vi "Obtain Doc Win ID.vi"(8 "error in (no error)":errorcluster, 11 "Document in":refnum<class "Document.lvclass">) -> (0 "error out":errorcluster, 3 "Document out":refnum<class "Document.lvclass">)   [LabVIEW 2016, in "Document.lvclass"]
uses:
  Document.lvclass
  Document.lvclass/Document.ctl
  user32.dll
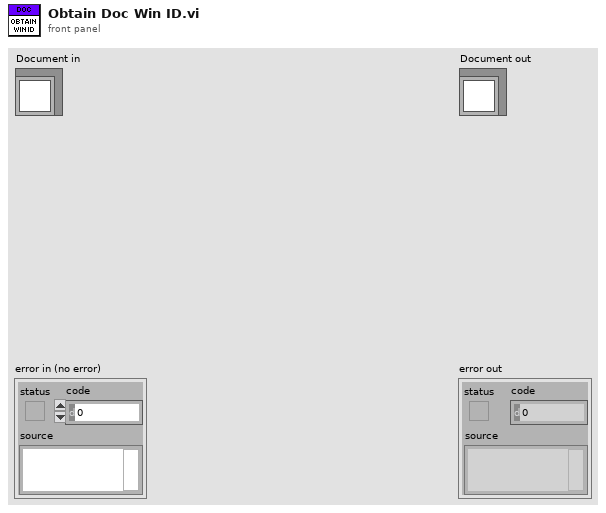
[diagram p1: front panel]
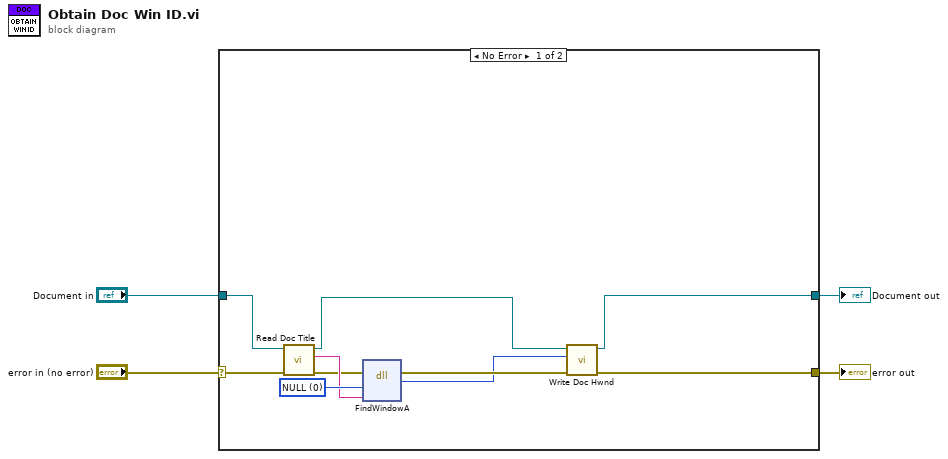
[diagram p0: block diagram]
diagram:
  n1 = case shown="No Error" "error in (no error)" {
    selector: "error in (no error)" -> [w8 w16]
    tunnel: [w7 w16] -> w3
    tunnel: [w5 w15] -> w1
    tunnel: "Document in" -> [w6 w15]
    frame No Error {
      w14 = 0 items=["NULL"]
      n2 = call "Read Doc Title.vi"("error in (no error)"=w8, "Document in"=w6) -> ("error out"=w10:errorcluster, "Doc Name"=w11:string, "Document out"=w9:refnum<class "Document.lvclass">)  [unwired: 7 in]
      n3 = dll-call lib="user32.dll" fn="FindWindowA"(error in=w10, "lpzsClassName"=w14, "lpzsWindowName"=w11) -> (error out=w13:errorcluster, "hwnd"=w12:u32)  [unwired: 4 in, 1 out]
      n4 = call "Write Doc Hwnd.vi"("error in (no error)"=w13, "Child Hwnd"=w12, "Document in"=w9) -> ("error out"=w7:errorcluster, "Document out"=w5:refnum<class "Document.lvclass">)  [unwired: 7 in]
    }
    frame Error {
    }
  }
  "error out" <- w3
  "Document out" <- w1
